vi "InjA-Image-RT.vi"() -> ()   [LabVIEW 2016]
uses:
  Common-Control/Cryo Readback.ctl
  Common-Control/Aperture states.ctl
  Common-Control/Faraday cup states.ctl
  Common-Control/GV states.ctl
  Common-Control/GP307 cluster.ctl
  <vilib>/userdefined/High Color/nirio_resource_hc.ctl
  Common-Control/Glassman Control.ctl
  <vilib>/FPGAPlugInAG/cRIO-9074/niLvFpga_Open_cRIO-9074.vi
  <vilib>/Utility/error.llb/Error Cluster From Error Code.vi
  <vilib>/rvi/errors/niLvFpgaAdjustHostInterfaceError.vi
  <vilib>/functionblocks/Control/PID/PID.vi
  <vilib>/rvi/interface/nirviOpenFPGA/nirviOpenFPGA.xnode
  FPGA Bitfiles/Controlsoftware2_FPGATarget_InjFPGA_-aTnSXeY2bA.lvbitx
  InjA-Image-FPGA.vi
  <vilib>/rvi/interface/nirviReadWriteControl/nirviReadWriteControl.xnode
  Common-Control/Faraday Cup Readback.ctl
  Common-Control/Aperture Readback.ctl
  Common-Control/Gate Valve Readback.ctl
  <vilib>/functionblocks/FB Core/FB Core.xnode
  <vilib>/functionblocks/FB Property/FB Overlay DBL.ctl
  <vilib>/functionblocks/NI_FunctionBlock Libraries.lvlib
  NiFpgaLv.dll
panel:
  out "Injector A Vac Interlock Bypass":bool
  out "Injector A Vac Interlock":bool
  out "Error Reporter":errorcluster
  in  "Tab Control":T1(tab)
  out "X-I":fxp<+/-,16,5>=1.28955078125
  out "X- V":fxp<+/-,16,5>=5.3388671875
  out "X+ I":fxp<+/-,16,5>=1.1064453125
  out "X+ V":fxp<+/-,16,5>=4.63671875
  out "Y+ V":fxp<+/-,16,5>=4.380859375
  out "Y+I":fxp<+/-,16,5>=1.068359375
  out "Y-V":fxp<+/-,16,5>=5.595703125
  out "Y-I":fxp<+/-,16,5>=1.36572265625
  out "Pre-acc V":fxp<+/-,16,5>=8.2509765625
  out "Pre-acc I":fxp<+/-,16,5>=2.544921875
  out "Einzel V":fxp<+/-,16,5>=7.4140625
  out "Einzel I":fxp<+/-,16,5>=1.6787109375
  out "X- Steerer Voltage Set":dbl
  out "X- Steerer HV Enable":bool
  out "X+ Steerer HV Enable":bool
  out "X+ Steerer Voltage Set":dbl
  out "Y- Steerer voltage set":dbl
  out "Y- Steerer HV Enable":bool
  out "Y+ Steerer HV Enable":bool
  out "Y+ Steerer voltage set":dbl
  out "Pre-Acc V set":dbl
  out "Pre-Acc HV Enable":bool
  out "Einzel HV Enable":bool
  out "Einzel V set":dbl
  in  "output low - switch":dbl
  in  "output high - switch":dbl=250.0
  out "Injector mag field set":dbl
  out "Injector mag field read 2":u8[](array[numeric])
  out "Injector mag field read":dbl
  out "Injector mag ps command":u8[](array[numeric])
  in  "derivative time (Td, min) - injector":dbl=0.01
  in  "integral time (Ti, min) - injector":dbl=0.01
  in  "proportional gain (Kc) - injector":dbl=10.0
  out "Injector mag command string":string
  out "Cryo Readback":T2
  out "Status":string
  out "On-time":string
  out "1st Stage Temp":string
  out "2nd Stage Temp":string
  out "Time since re-purge":string
  out "LowEnd Waist Vac Interlock":bool
  out "LowEnd Waist Vac Interlock bypass":bool
  out "Vac Interlock":bool
  out "Time since repurge":u8[](array[numeric])
  out "2nd stage temp":u8[](array[numeric])
  out "Cryo 1st stage temp":u8[](array[numeric])
  out "Cryo On-time":u8[](array[numeric])
  out "Cryo status":u8[](array[numeric])
  out "InjA Image Interlock bypass":bool
  out "Convectron 2":u8[](array[numeric])
  out "Ion Gauge 2":u8[](array[numeric])
  out "InjA Image Ion Gauge 1":dbl
  out "InjA Image Vac Cluster":T3
  out "InjA Image Convectron 1":dbl
  out "Convectron 1":u8[](array[numeric])
  out "Ion Gauge 1":u8[](array[numeric])
  out "Inj Image Aperture actuator":bool
  out "Inj Image FC actuator":bool
  out "Cryo Pump GV actuator":bool
  out "Beamline GV actuator":bool
  out "Inj Image Image  Aperture Position 2":T4
  out "Inj Image Image  Aperture Position":cluster{"IN sensor":bool, "OUT sensor":bool}
  out "Inj Image FC Status":T5
  out "Inj Image FC Position":cluster{"IN sensor":bool, "OUT sensor":bool}
  out "Beamline GV status":T6
  out "Beamline GV Position":T7
  out "Cryo Pump GV status":T6
  out "Cryo Pump GV Position":T7
  out "HV control loop error":errorcluster
  out "HV Readback loop error":errorcluster
  out "Injector Magnet error":errorcluster
  out "Cryo loop error":errorcluster
  out "GV Interlock loop error":errorcluster
  out "Acuator-Sensor loop error":errorcluster
  out "Vac cluster loop error":errorcluster
  in  "error in":errorcluster
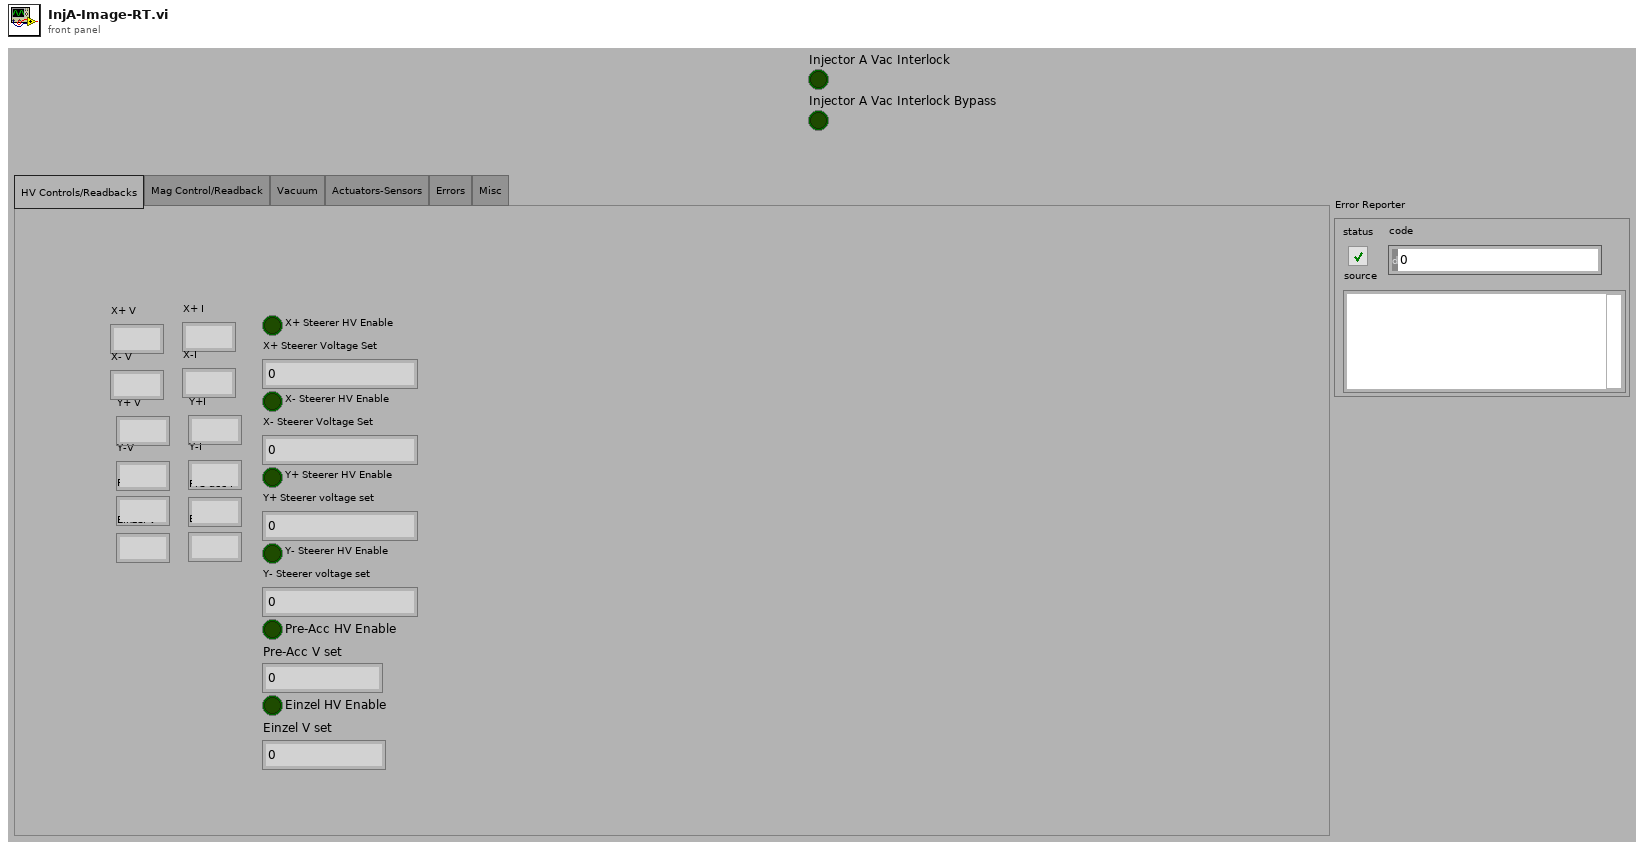
[diagram p1: front panel]
types:
  T1 = enum32{"HV Controls/Readbacks", "Mag Control/Readback", "Vacuum", "Actuators-Sensors", "Errors", "Misc"}
  T2 = typedef "Cryo Readback.ctl" = cluster{"Status":string, "On-time":string, "1st Stage Temp":string, "2nd Stage Temp":string, "Time since re-purge":string}
  T3 = typedef "GP307 cluster.ctl" = cluster{"Ion gauge 1":string, "Convectron  Gauge 1 ":string, "Ion Gauge 2":string, "Convectrom Gauge 2":string}
  T4 = typedef "Aperture states.ctl" = enum16{"Aperture status unclear", "Aperture in", "Aperture out"}
  T5 = typedef "Faraday cup states.ctl" = enum16{"FC status unclear", "FC in", "FC out"}
  T6 = typedef "GV states.ctl" = enum16{"status unclear", "closed", "open"}
  T7 = cluster{"OPEN sensor":bool, "Closed sensor":bool}
  T8 = typedef "nirio_resource_hc.ctl" = tag
  T9 = typedef "Faraday Cup Readback.ctl" = cluster{"IN sensor":bool, "OUT sensor":bool}
  T10 = typedef "Aperture Readback.ctl" = cluster{"IN sensor":bool, "OUT sensor":bool}
  T11 = typedef "Gate Valve Readback.ctl" = cluster{"OPEN sensor":bool, "Closed sensor":bool}
  T12 = typedef "Glassman Control.ctl" = cluster{"V-program":fxp<+/-,16,5>, "HV Enable":bool}
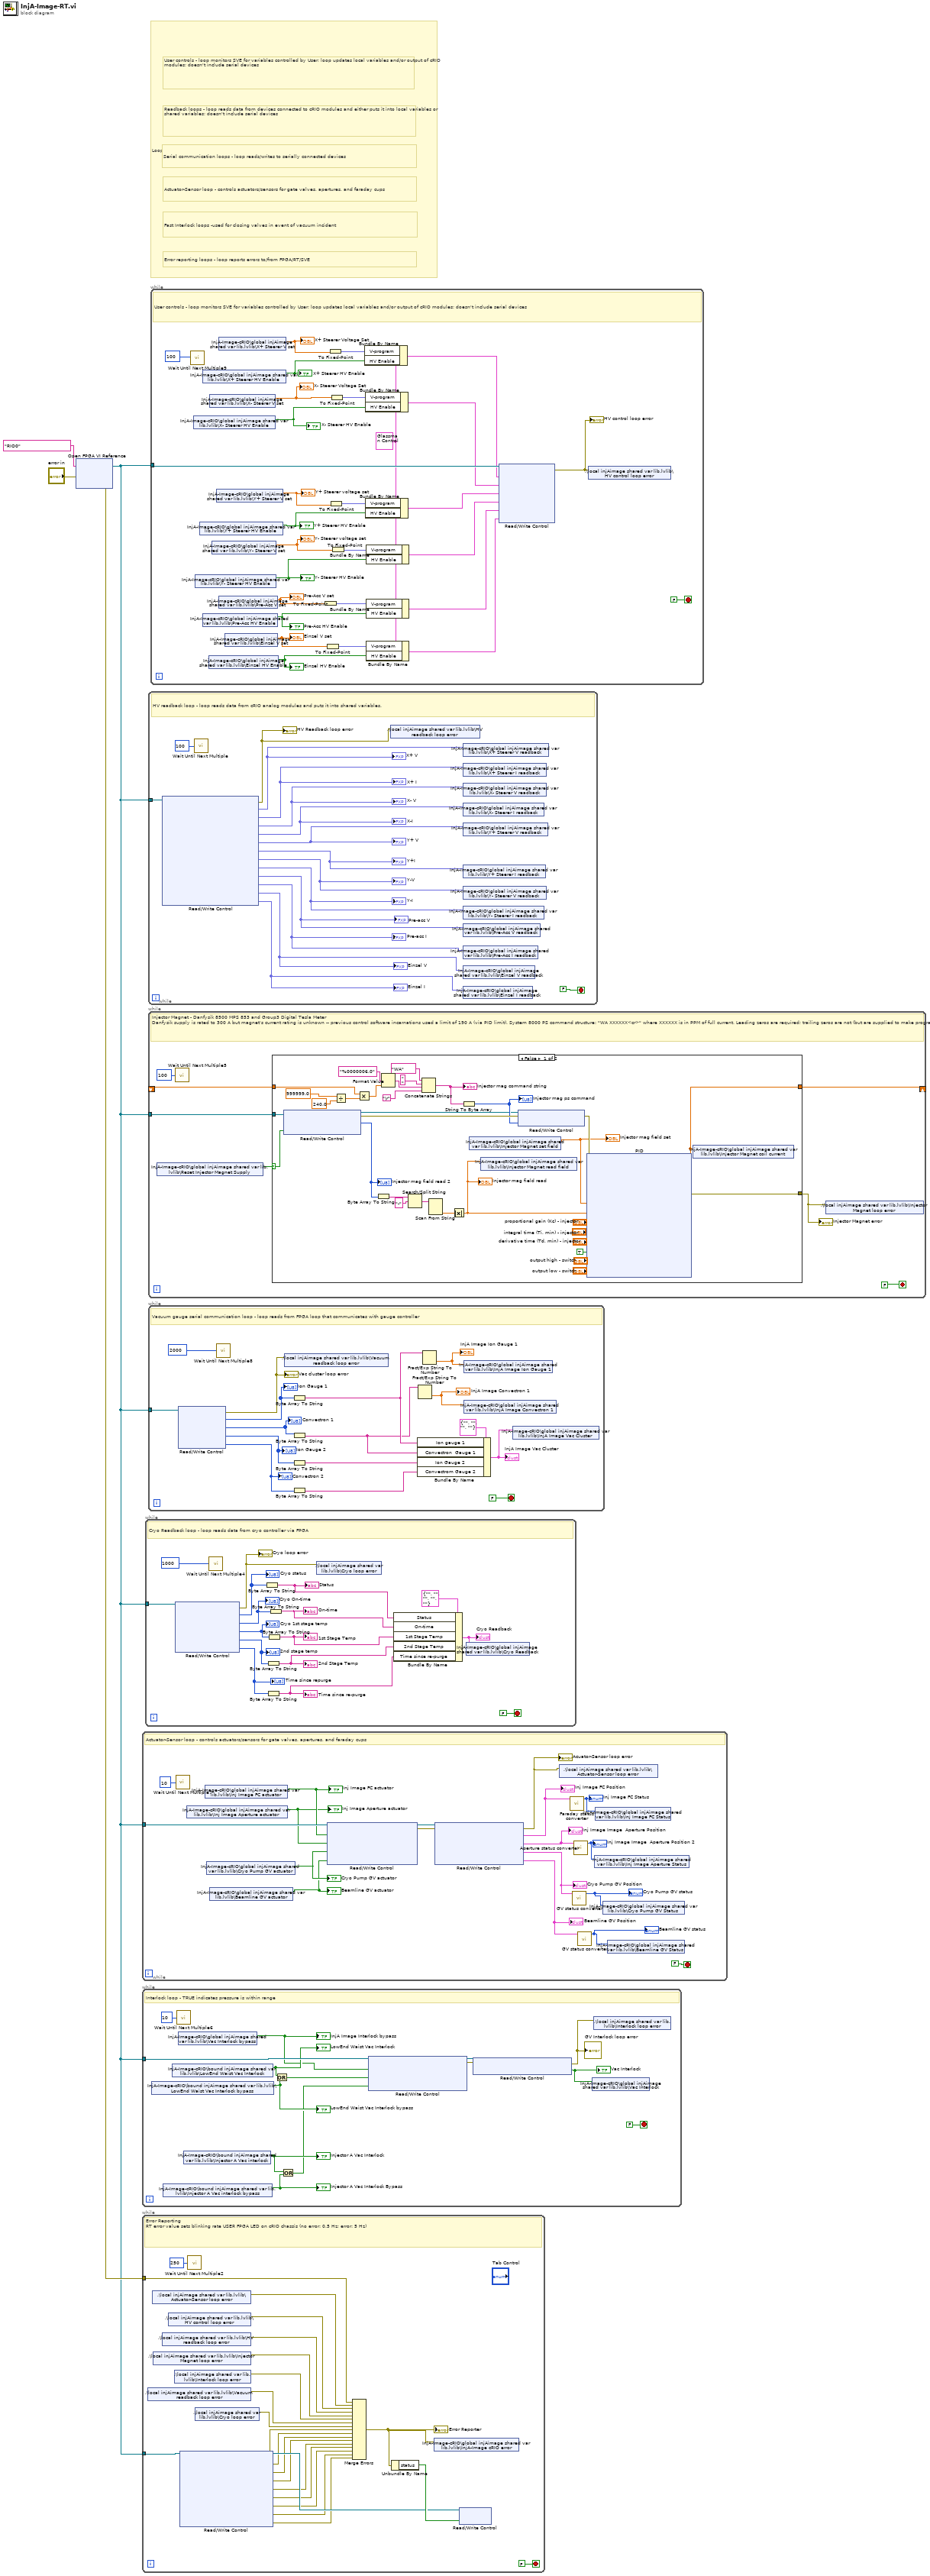
[diagram p0: block diagram]
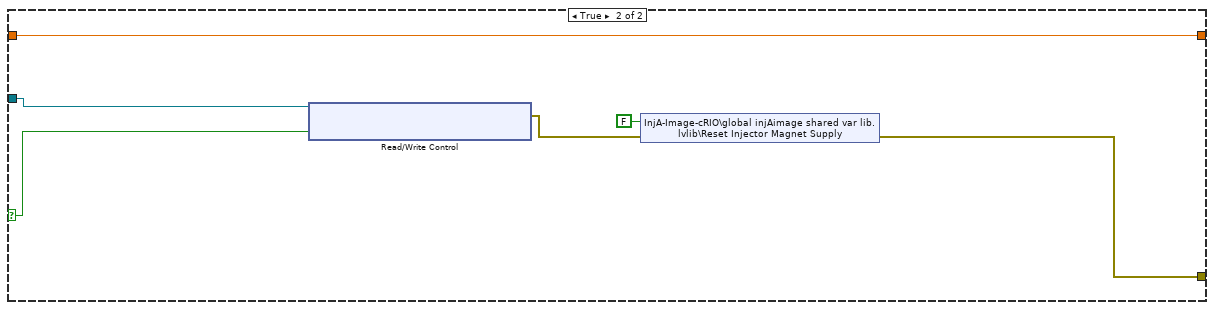
[diagram p2: hidden frame]
diagram:
  # "Serial communication loops - loop reads/writes to serially connected devices"
  # "Actuator-Sensor loop - controls actuators/sensors for gate valves, apertures, and faraday cups"
  # "Fast Interlock loops -used for closing valves in event of vacuum incident"
  # "Error reporting loops - loop reports errors to/from FPGA/RT/SVE"
  # "Readback loops - loop reads data from devices connected to cRIO modules and either puts it into local variables or shared variables; doesn't include serial devices"
  # "User controls - loop monitors SVE for variables controlled by User; loop updates local variables and/or output of cRIO modules; doesn't include serial devices"
  # "Loop legend - loops are color coded by responsibility"
  n1 = xnode "Open FPGA VI Reference"("error in"="error in", "resource name"=T8 "RIO0") -> ("FPGA VI Reference Out"=w1:refnum<k20>, "error out"=w2:errorcluster)
  n2 = while {
    tunnel: w1 -> [w22]
    stop <- FALSE stop-if-true
    # "Actuator-Sensor loop - controls actuators/sensors for gate valves, apertures, and faraday cups"
    n3 = call "Wait Until Next Multiple7"("Count(mSec)"=u32 10) -> ()  [unwired: 1 out]
    n4 = shared-variable "InjA-Image-cRIO\\global injAimage shared var lib.lvlib\\Inj Image Aperture actuator"() -> (w8:bool)  [unwired: 1 in, 1 out]
    "Inj Image Aperture actuator" <- w8
    n5 = shared-variable "InjA-Image-cRIO\\global injAimage shared var lib.lvlib\\Inj Image FC actuator"() -> (w9:bool)  [unwired: 1 in, 1 out]
    "Inj Image FC actuator" <- w9
    n6 = shared-variable "InjA-Image-cRIO\\global injAimage shared var lib.lvlib\\Cryo Pump GV actuator"() -> (w11:bool)  [unwired: 1 in, 1 out]
    "Cryo Pump GV actuator" <- w11
    n7 = shared-variable "InjA-Image-cRIO\\global injAimage shared var lib.lvlib\\Beamline GV actuator"() -> (w10:bool)  [unwired: 1 in, 1 out]
    "Beamline GV actuator" <- w10
    n8 = xnode "Read/Write Control"("FPGA VI Reference In"=w22, "Inj Image FC Actuator"=w9, "Inj Image Aperture Actuator"=w8, "Cryo Pump GV Actuator"=w11, "Beamline GV Actuator"=w10) -> ("FPGA VI Reference Out"=w20:refnum<k20>, "error out"=w18:errorcluster)  [unwired: 1 in]
    n9 = xnode "Read/Write Control"("FPGA VI Reference In"=w20, "error in"=w18) -> ("error out"=w12:errorcluster, "Inj Image FC Position"=w14:T9, "Inj Image Aperture Position"=w13:T10, "Cryo Pump GV Status"=w17:T11, "Beamline GV Status"=w16:T11)  [unwired: 1 out]
    "Cryo Pump GV Position" <- w17
    "Beamline GV Position" <- w16
    "Inj Image FC Position" <- w14
    "Inj Image Image  Aperture Position" <- w13
    "Acuator-Sensor loop error" <- w12
    n10 = shared-variable ".\\local injAimage shared var lib.lvlib\\Actuator-Sensor loop error"(w12) -> ()  [unwired: 1 in, 1 out]
    n11 = call "Faraday status converter.vi"("FC Position"=w14) -> ("FC Status"=w15:T5)  [unwired: 10 in]
    "Inj Image FC Status" <- w15
    n12 = call "GV status converter.vi"("Gate Valve"=w17) -> ("GV Status"=w6:T6)  [unwired: 10 in]
    "Cryo Pump GV status" <- w6
    n13 = call "Aperture status converter.vi"("Aperture Position"=w13) -> ("Aperture Status"=w5:T4)  [unwired: 10 in]
    "Inj Image Image  Aperture Position 2" <- w5
    n14 = call "GV status converter.vi"("Gate Valve"=w16) -> ("GV Status"=w7:T6)  [unwired: 10 in]
    "Beamline GV status" <- w7
    n15 = shared-variable "InjA-Image-cRIO\\global injAimage shared var lib.lvlib\\Inj Image Aperture Status"(w5) -> ()  [unwired: 1 in, 1 out]
    n16 = shared-variable "InjA-Image-cRIO\\global injAimage shared var lib.lvlib\\Inj Image FC Status"(w15) -> ()  [unwired: 1 in, 1 out]
    n17 = shared-variable "InjA-Image-cRIO\\global injAimage shared var lib.lvlib\\Cryo Pump GV Status"(w6) -> ()  [unwired: 1 in, 1 out]
    n18 = shared-variable "InjA-Image-cRIO\\global injAimage shared var lib.lvlib\\Beamline GV Status"(w7) -> ()  [unwired: 1 in, 1 out]
  }
  n19 = while {
    tunnel: w1 -> [w36]
    stop <- FALSE stop-if-true
    # "Interlock loop - TRUE indicates pressure is within range"
    n20 = shared-variable "InjA-Image-cRIO\\bound injAimage shared var lib.lvlib\\LowEnd Waist Vac Interlock bypass"() -> (w30:bool)  [unwired: 1 in, 1 out]
    "LowEnd Waist Vac Interlock bypass" <- w30
    n21 = shared-variable "InjA-Image-cRIO\\bound injAimage shared var lib.lvlib\\Injector A Vac interlock bypass"() -> (w25:bool)  [unwired: 1 in, 1 out]
    "Injector A Vac Interlock Bypass" <- w25
    n22 = shared-variable "InjA-Image-cRIO\\bound injAimage shared var lib.lvlib\\LowEnd Waist Vac Interlock"() -> (w28:bool)  [unwired: 1 in, 1 out]
    "LowEnd Waist Vac Interlock" <- w28
    n23 = call "Wait Until Next Multiple6"("Count(mSec)"=u32 10) -> ()  [unwired: 1 out]
    n24 = shared-variable "InjA-Image-cRIO\\global injAimage shared var lib.lvlib\\Vac Interlock bypass"() -> (w23:bool)  [unwired: 1 in, 1 out]
    "InjA Image Interlock bypass" <- w23
    n25 = shared-variable "InjA-Image-cRIO\\bound injAimage shared var lib.lvlib\\Injector A Vac interlock"() -> (w26:bool)  [unwired: 1 in, 1 out]
    "Injector A Vac Interlock" <- w26
    n26 = Or(x=w28, y=w30) -> (x .or. y?=w29:bool)
    n27 = Or(x=w26, y=w25) -> (x .or. y?=w24:bool)
    n28 = xnode "Read/Write Control"("FPGA VI Reference In"=w36, "Vac Interlock Bypass"=w23, "LowEnd Waist Vac Interlock"=w29, "InjectorA Vac Interlock"=w24) -> ("FPGA VI Reference Out"=w35:refnum<k20>, "error out"=w34:errorcluster)  [unwired: 1 in]
    n29 = xnode "Read/Write Control"("FPGA VI Reference In"=w35, "error in"=w34) -> ("error out"=w33:errorcluster, "Vac Interlock"=w27:bool)  [unwired: 1 out]
    "GV Interlock loop error" <- w33
    "Vac Interlock" <- w27
    n30 = shared-variable "InjA-Image-cRIO\\global injAimage shared var lib.lvlib\\Vac Interlock"(w27) -> ()  [unwired: 1 in, 1 out]
    n31 = shared-variable ".\\local injAimage shared var lib.lvlib\\Interlock loop error"(w33) -> ()  [unwired: 1 in, 1 out]
  }
  n32 = while {
    tunnel: w1 -> [w52]
    tunnel: w2 -> [w42]
    stop <- FALSE stop-if-true
    # "Error Reporting\nRT error value sets blinking rate USER FPGA LED on cRIO chassis (no error: 0.5 Hz; error: 5 Hz)"
    n33 = shared-variable ".\\local injAimage shared var lib.lvlib\\Vacuum readback loop error"() -> (w54:errorcluster)  [unwired: 1 in, 1 out]
    n34 = shared-variable ".\\local injAimage shared var lib.lvlib\\Actuator-Sensor loop error"() -> (w40:errorcluster)  [unwired: 1 in, 1 out]
    n35 = shared-variable ".\\local injAimage shared var lib.lvlib\\Injector Magnet loop error"() -> (w56:errorcluster)  [unwired: 1 in, 1 out]
    n36 = shared-variable ".\\local injAimage shared var lib.lvlib\\HV readback loop error"() -> (w57:errorcluster)  [unwired: 1 in, 1 out]
    n37 = shared-variable ".\\local injAimage shared var lib.lvlib\\HV control loop error"() -> (w41:errorcluster)  [unwired: 1 in, 1 out]
    n38 = shared-variable ".\\local injAimage shared var lib.lvlib\\Interlock loop error"() -> (w55:errorcluster)  [unwired: 1 in, 1 out]
    n39 = xnode "Read/Write Control"("FPGA VI Reference In"=w52) -> ("FPGA VI Reference Out"=w51:refnum<k20>, "error out"=w50:errorcluster, "GV Interlock loop error"=w49:errorcluster, "Actuator-Sensor Loop error"=w48:errorcluster, "Injector Hall Probe error"=w47:errorcluster, "Injector Magnet control error"=w46:errorcluster, "Vac readback loop error"=w45:errorcluster, "HV control loop error"=w44:errorcluster, "Cryo pump error"=w38:errorcluster, "HV Readback loop"=w37:errorcluster)  [unwired: 1 in]
    n40 = call "Wait Until Next Multiple2"("Count(mSec)"=u32 250 ("millisecond multiple")) -> ()  [unwired: 1 out]
    n41 = shared-variable ".\\local injAimage shared var lib.lvlib\\Cryo loop error"() -> (w53:errorcluster)  [unwired: 1 in, 1 out]
    n42 = Merge Errors(w42, w40, w41, w57, w56, w55, w54, w53, w50, w49, w48, w47, w46, w45, w44, w38, w37) -> (w59:errorcluster)
    "Error Reporter" <- w59
    n43 = Unbundle By Name(w59) -> ("status"=w58:bool)
    n44 = shared-variable "InjA-Image-cRIO\\global injAimage shared var lib.lvlib\\InjA-Image cRIO error"(w59) -> ()  [unwired: 1 in, 1 out]
    n45 = xnode "Read/Write Control"("FPGA VI Reference In"=w51, "RT error"=w58) -> ()  [unwired: 1 in, 2 out]
  }
  n46 = while {
    tunnel: w1 -> [w74]
    stop <- FALSE stop-if-true
    # "Cryo Readback loop - loop reads data from cryo controller via FPGA"
    n47 = xnode "Read/Write Control"("FPGA VI Reference In"=w74) -> ("error out"=w60:errorcluster, "Cryo status"=w71:u8[], "Cryo On-time"=w72:u8[], "1st stage temp"=w73:u8[], "2nd stage temp"=w70:u8[], "Time since repurge"=w69:u8[])  [unwired: 1 in, 1 out]
    "Cryo status" <- w71
    "Cryo On-time" <- w72
    "Cryo 1st stage temp" <- w73
    "Cryo loop error" <- w60
    "2nd stage temp" <- w70
    "Time since repurge" <- w69
    n48 = call "Wait Until Next Multiple4"("Count(mSec)"=u32 1000 ("millisecond multiple")) -> ()  [unwired: 1 out]
    n49 = Byte Array To String(unsigned byte array=w71) -> (string=w65:string)
    "Status" <- w65
    n50 = Byte Array To String(unsigned byte array=w70) -> (string=w62:string)
    "2nd Stage Temp" <- w62
    n51 = Byte Array To String(unsigned byte array=w69) -> (string=w61:string)
    "Time since re-purge" <- w61
    n52 = Byte Array To String(unsigned byte array=w73) -> (string=w63:string)
    "1st Stage Temp" <- w63
    n53 = Byte Array To String(unsigned byte array=w72) -> (string=w64:string)
    "On-time" <- w64
    n54 = shared-variable ".\\local injAimage shared var lib.lvlib\\Cryo loop error"(w60) -> ()  [unwired: 1 in, 1 out]
    n55 = Bundle By Name(cluster=T2 {"Status"="", "On-time"="", "1st Stage Temp"="", "2nd Stage Temp"="", "Time since re-purge"=""} ("Cryo Readback"), "Status"=w65, "On-time"=w64, "1st Stage Temp"=w63, "2nd Stage Temp"=w62, "Time since re-purge"=w61) -> (w67:T2)
    "Cryo Readback" <- w67
    n56 = shared-variable "InjA-Image-cRIO\\global injAimage shared var lib.lvlib\\Cryo Readback"(w67) -> ()  [unwired: 1 in, 1 out]
  }
  n57 = while {
    shift-right: [w78] -> _
    shift-left: _ -> [w80]
    tunnel: w1 -> [w81]
    stop <- FALSE stop-if-true
    # "Injector Magnet - Danfysik 8500 MPS 853 and Group3 Digital Tesla Meter\nDanfysik supply is rated to 300 A but magnet's current rating is unknown -- previous control software incarnations used a limit of 190 A (via PID limit). System 8000 PS command structure: \"WA XXXXXX<cr>\" where XXXXXX is in PPM of full current. Leading zeros are required; trailing zeros are not (but are supplied to make programming easier)"
    n58 = shared-variable "InjA-Image-cRIO\\global injAimage shared var lib.lvlib\\Reset Injector Magnet Supply"() -> (w77:bool)  [unwired: 1 in, 1 out]
    n59 = call "Wait Until Next Multiple5"("Count(mSec)"=u32 100 ("millisecond multiple")) -> ()  [unwired: 1 out]
    n60 = case shown="False" w77 {
      selector: w77 -> [w85 w184]
      tunnel: w81 -> [w101 w186]
      tunnel: w80 -> [w97 w185]
      tunnel: [w86 w185] -> w78
      tunnel: [w84 w181] -> w76
      frame False {
        n61 = xnode "Read/Write Control"("FPGA VI Reference In"=w101, "Inj Magnet Reset"=w85) -> ("FPGA VI Reference Out"=w95:refnum<k20>, "error out"=w100:errorcluster, "Injector Mag Field read"=w96:u8[])  [unwired: 1 in]
        "Injector mag field read 2" <- w96
        n62 = Divide(x=999999.0 ("y"), y=240.0) -> (x/y=w89:dbl)
        n63 = Multiply(x=w97, y=w89) -> (x*y=w110:dbl)
        n64 = Byte Array To String(unsigned byte array=w96) -> (string=w107:string)
        n65 = Format Value(format string="%0000006.0", value (0)=w110) -> (output string=w113:string)  [unwired: 1 out]
        n66 = Search/Split String(string=w107, search string/char (-)="-") -> (match + rest of string=w98:string)  [unwired: 3 out]
        n67 = Concatenate Strings("WA", " ", w113, "\r") -> (w114:string)
        "Injector mag command string" <- w114
        n68 = Scan From String(input string=w98) -> (output 1=w106:dbl)  [unwired: 3 in, 4 out]
        n69 = Absolute Value(x=w106) -> (abs(x)=w83:dbl)
        "Injector mag field read" <- w83
        n70 = String To Byte Array(string=w114) -> (unsigned byte array=w99:u8[])
        "Injector mag ps command" <- w99
        n71 = shared-variable "InjA-Image-cRIO\\global injAimage shared var lib.lvlib\\Injector Magnet set field"() -> (w87:dbl)  [unwired: 1 in, 1 out]
        "Injector mag field set" <- w87
        n72 = shared-variable "InjA-Image-cRIO\\global injAimage shared var lib.lvlib\\Injector Magnet read field"(w83) -> ()  [unwired: 1 in, 1 out]
        n73 = xnode "Read/Write Control"("FPGA VI Reference In"=w95, "error in"=w100, "Injector Magnet Set"=w99) -> ("error out"=w94:errorcluster)  [unwired: 1 out]
        n74 = xnode "PID"("error in"=w94, "setpoint"=w87, "process variable"=w83, "proportional gain (Kc)"="proportional gain (Kc) - injector", "integral time (Ti, min)"="integral time (Ti, min) - injector", "derivative time (Td, min)"="derivative time (Td, min) - injector", "auto? (T)"=TRUE, "output high"="output high - switch", "output low"="output low - switch") -> ("error out"=w84:errorcluster, "output"=w86:dbl)
        n75 = shared-variable "InjA-Image-cRIO\\global injAimage shared var lib.lvlib\\Injector Magnet coil current"(w86) -> ()  [unwired: 1 in, 1 out]
      }
      frame True {
        n76 = xnode "Read/Write Control"("FPGA VI Reference In"=w186, "Inj Magnet Reset"=w184) -> ("error out"=w182:errorcluster)  [unwired: 1 in, 1 out]
        n77 = shared-variable "InjA-Image-cRIO\\global injAimage shared var lib.lvlib\\Reset Injector Magnet Supply"(FALSE ("Reset Injector Magnet Supply"), error in=w182) -> (error out=w181:errorcluster)
      }
    }
    "Injector Magnet error" <- w76
    n78 = shared-variable ".\\local injAimage shared var lib.lvlib\\Injector Magnet loop error"(w76) -> ()  [unwired: 1 in, 1 out]
  }
  n79 = while {
    tunnel: w1 -> [w197]
    stop <- FALSE stop-if-true
    # "Vacuum gauge serial communication loop - loop reads from FPGA loop that communicates with gauge controller"
    n80 = xnode "Read/Write Control"("FPGA VI Reference In"=w197) -> ("error out"=w192:errorcluster, "Ion gauge 1"=w198:u8[], "Convectron 1"=w194:u8[], "Ion gauge 2"=w199:u8[], "Convectron 2"=w200:u8[])  [unwired: 1 in, 1 out]
    "Ion Gauge 1" <- w198
    "Convectron 1" <- w194
    "Ion Gauge 2" <- w199
    "Convectron 2" <- w200
    "Vac cluster loop error" <- w192
    n81 = call "Wait Until Next Multiple8"("Count(mSec)"=u32 2000 ("millisecond multiple")) -> ()  [unwired: 1 out]
    n82 = shared-variable ".\\local injAimage shared var lib.lvlib\\Vacuum readback loop error"(w192) -> ()  [unwired: 1 in, 1 out]
    n83 = Byte Array To String(unsigned byte array=w198) -> (string=w195:string)
    n84 = Byte Array To String(unsigned byte array=w194) -> (string=w193:string)
    n85 = Byte Array To String(unsigned byte array=w199) -> (string=w201:string)
    n86 = Byte Array To String(unsigned byte array=w200) -> (string=w202:string)
    n87 = Bundle By Name(cluster=T3 {"Ion gauge 1"="", "Convectron  Gauge 1 "="", "Ion Gauge 2"="", "Convectrom Gauge 2"=""} ("Ion gauge cluster control"), "Ion gauge 1"=w195, "Convectron  Gauge 1"=w193, "Ion Gauge 2"=w201, "Convectrom Gauge 2"=w202) -> (w189:T3)
    "InjA Image Vac Cluster" <- w189
    n88 = Fract/Exp String To Number(string=w193) -> (number=w188:dbl)  [unwired: 3 in, 1 out]
    "InjA Image Convectron 1" <- w188
    n89 = Fract/Exp String To Number(string=w195) -> (number=w187:dbl)  [unwired: 3 in, 1 out]
    "InjA Image Ion Gauge 1" <- w187
    n90 = shared-variable "InjA-Image-cRIO\\global injAimage shared var lib.lvlib\\InjA Image Ion Gauge 1"(w187) -> ()  [unwired: 1 in, 1 out]
    n91 = shared-variable "InjA-Image-cRIO\\global injAimage shared var lib.lvlib\\InjA Image Convectron 1"(w188) -> ()  [unwired: 1 in, 1 out]
    n92 = shared-variable "InjA-Image-cRIO\\global injAimage shared var lib.lvlib\\InjA Image Vac Cluster"(w189) -> ()  [unwired: 1 in, 1 out]
  }
  n93 = while {
    tunnel: w1 -> [w204]
    stop <- FALSE stop-if-true
    # "HV readback loop - loop reads data from cRIO analog modules and puts it into shared variables."
    n94 = xnode "Read/Write Control"("FPGA VI Reference In"=w204) -> ("error out"=w203:errorcluster, "X+ Steerer Monitor.I-monitor"=w216:fxp<+/-,16,5>, "X+ Steerer Monitor.V-monitor"=w215:fxp<+/-,16,5>, "X- Steerer Monitor.I-monitor"=w214:fxp<+/-,16,5>, "X- Steerer Monitor.V-monitor"=w213:fxp<+/-,16,5>, "Y+ Steerer Monitor.I-monitor"=w212:fxp<+/-,16,5>, "Y+ Steerer Monitor.V-monitor"=w205:fxp<+/-,16,5>, "Y- Steerer Monitor.I-monitor"=w206:fxp<+/-,16,5>, "Y- Steerer Monitor.V-monitor"=w207:fxp<+/-,16,5>, "Pre-Acc Monitor.I-monitor"=w208:fxp<+/-,16,5>, "Pre-Acc Monitor.V-monitor"=w209:fxp<+/-,16,5>, "Einzel Monitor.I-monitor"=w210:fxp<+/-,16,5>, "Einzel Monitor.V-monitor"=w211:fxp<+/-,16,5>)  [unwired: 1 in, 1 out]
    "Y+ V" <- w212
    "Y+I" <- w205
    "Y-V" <- w206
    "Y-I" <- w207
    "Pre-acc V" <- w208
    "Pre-acc I" <- w209
    "Einzel V" <- w210
    "Einzel I" <- w211
    "X+ V" <- w216
    "X+ I" <- w215
    "X- V" <- w214
    "X-I" <- w213
    "HV Readback loop error" <- w203
    n95 = call "Wait Until Next Multiple"("Count(mSec)"=u32 100) -> ()  [unwired: 1 out]
    n96 = shared-variable ".\\local injAimage shared var lib.lvlib\\HV readback loop error"(w203) -> ()  [unwired: 1 in, 1 out]
    n97 = shared-variable "InjA-Image-cRIO\\global injAimage shared var lib.lvlib\\X+ Steerer V readback"(w216) -> ()  [unwired: 1 in, 1 out]
    n98 = shared-variable "InjA-Image-cRIO\\global injAimage shared var lib.lvlib\\X+ Steerer I readback"(w215) -> ()  [unwired: 1 in, 1 out]
    n99 = shared-variable "InjA-Image-cRIO\\global injAimage shared var lib.lvlib\\X- Steerer V readback"(w214) -> ()  [unwired: 1 in, 1 out]
    n100 = shared-variable "InjA-Image-cRIO\\global injAimage shared var lib.lvlib\\X- Steerer I readback"(w213) -> ()  [unwired: 1 in, 1 out]
    n101 = shared-variable "InjA-Image-cRIO\\global injAimage shared var lib.lvlib\\Y+ Steerer V readback"(w212) -> ()  [unwired: 1 in, 1 out]
    n102 = shared-variable "InjA-Image-cRIO\\global injAimage shared var lib.lvlib\\Y+ Steerer I readback"(w205) -> ()  [unwired: 1 in, 1 out]
    n103 = shared-variable "InjA-Image-cRIO\\global injAimage shared var lib.lvlib\\Y- Steerer V readback"(w206) -> ()  [unwired: 1 in, 1 out]
    n104 = shared-variable "InjA-Image-cRIO\\global injAimage shared var lib.lvlib\\Y- Steerer I readback"(w207) -> ()  [unwired: 1 in, 1 out]
    n105 = shared-variable "InjA-Image-cRIO\\global injAimage shared var lib.lvlib\\Pre-Acc V readback"(w208) -> ()  [unwired: 1 in, 1 out]
    n106 = shared-variable "InjA-Image-cRIO\\global injAimage shared var lib.lvlib\\Pre-Acc I readback"(w209) -> ()  [unwired: 1 in, 1 out]
    n107 = shared-variable "InjA-Image-cRIO\\global injAimage shared var lib.lvlib\\Einzel V readback"(w210) -> ()  [unwired: 1 in, 1 out]
    n108 = shared-variable "InjA-Image-cRIO\\global injAimage shared var lib.lvlib\\Einzel I readback"(w211) -> ()  [unwired: 1 in, 1 out]
  }
  n109 = while {
    tunnel: w1 -> [w247]
    stop <- FALSE stop-if-true
    w227 = T12 {"V-program"=0.0, "HV Enable"=FALSE} ("Glassman Control")
    # "User controls - loop monitors SVE for variables controlled by User; loop updates local variables and/or output of cRIO modules; doesn't include serial devices"
    n110 = call "Wait Until Next Multiple9"("Count(mSec)"=u32 100 ("millisecond multiple")) -> ()  [unwired: 1 out]
    n111 = shared-variable "InjA-Image-cRIO\\global injAimage shared var lib.lvlib\\X- Steerer HV Enable"() -> (w233:bool)  [unwired: 1 in, 1 out]
    "X- Steerer HV Enable" <- w233
    n112 = shared-variable "InjA-Image-cRIO\\global injAimage shared var lib.lvlib\\Y- Steerer HV Enable"() -> (w229:bool)  [unwired: 1 in, 1 out]
    "Y- Steerer HV Enable" <- w229
    n113 = shared-variable "InjA-Image-cRIO\\global injAimage shared var lib.lvlib\\Y+ Steerer HV Enable"() -> (w231:bool)  [unwired: 1 in, 1 out]
    "Y+ Steerer HV Enable" <- w231
    n114 = shared-variable "InjA-Image-cRIO\\global injAimage shared var lib.lvlib\\X+ Steerer HV Enable"() -> (w236:bool)  [unwired: 1 in, 1 out]
    "X+ Steerer HV Enable" <- w236
    n115 = shared-variable "InjA-Image-cRIO\\global injAimage shared var lib.lvlib\\Pre-Acc HV Enable"() -> (w221:bool)  [unwired: 1 in, 1 out]
    "Pre-Acc HV Enable" <- w221
    n116 = shared-variable "InjA-Image-cRIO\\global injAimage shared var lib.lvlib\\Einzel HV Enable"() -> (w223:bool)  [unwired: 1 in, 1 out]
    "Einzel HV Enable" <- w223
    n117 = shared-variable "InjA-Image-cRIO\\global injAimage shared var lib.lvlib\\X- Steerer V set"() -> (w234:dbl)  [unwired: 1 in, 1 out]
    "X- Steerer Voltage Set" <- w234
    n118 = shared-variable "InjA-Image-cRIO\\global injAimage shared var lib.lvlib\\Y- Steerer V set"() -> (w230:dbl)  [unwired: 1 in, 1 out]
    "Y- Steerer voltage set" <- w230
    n119 = shared-variable "InjA-Image-cRIO\\global injAimage shared var lib.lvlib\\Y+ Steerer V set"() -> (w232:dbl)  [unwired: 1 in, 1 out]
    "Y+ Steerer voltage set" <- w232
    n120 = shared-variable "InjA-Image-cRIO\\global injAimage shared var lib.lvlib\\X+ Steerer V set"() -> (w235:dbl)  [unwired: 1 in, 1 out]
    "X+ Steerer Voltage Set" <- w235
    n121 = shared-variable "InjA-Image-cRIO\\global injAimage shared var lib.lvlib\\Pre-Acc V set"() -> (w222:dbl)  [unwired: 1 in, 1 out]
    "Pre-Acc V set" <- w222
    n122 = shared-variable "InjA-Image-cRIO\\global injAimage shared var lib.lvlib\\Einzel V set"() -> (w224:dbl)  [unwired: 1 in, 1 out]
    "Einzel V set" <- w224
    n123 = To Fixed-Point(number=w222) -> (fixed-point=w220:fxp<+/-,16,5>)  [unwired: 1 in]
    n124 = To Fixed-Point(number=w224) -> (fixed-point=w219:fxp<+/-,16,5>)  [unwired: 1 in]
    n125 = To Fixed-Point(number=w235) -> (fixed-point=w240:fxp<+/-,20,5>)  [unwired: 1 in]
    n126 = To Fixed-Point(number=w232) -> (fixed-point=w244:fxp<+/-,16,5>)  [unwired: 1 in]
    n127 = To Fixed-Point(number=w234) -> (fixed-point=w239:fxp<+/-,16,5>)  [unwired: 1 in]
    n128 = To Fixed-Point(number=w230) -> (fixed-point=w243:fxp<+/-,16,5>)  [unwired: 1 in]
    n129 = Bundle By Name(cluster=w227, "V-program"=w240, "HV Enable"=w236) -> (w237:T12)
    n130 = Bundle By Name(cluster=w227, "V-program"=w239, "HV Enable"=w233) -> (w238:T12)
    n131 = Bundle By Name(cluster=w227, "V-program"=w244, "HV Enable"=w231) -> (w241:T12)
    n132 = Bundle By Name(cluster=w227, "V-program"=w243, "HV Enable"=w229) -> (w242:T12)
    n133 = Bundle By Name(cluster=w227, "V-program"=w220, "HV Enable"=w221) -> (w226:T12)
    n134 = Bundle By Name(cluster=w227, "V-program"=w219, "HV Enable"=w223) -> (w225:T12)
    n135 = xnode "Read/Write Control"("FPGA VI Reference In"=w247, "X+ Steerer V set"=w237, "X- Steerer V set"=w238, "Y+ Steerer V set"=w241, "Y- Steerer V set"=w242, "Pre-Acc V set"=w226, "Einzel V set"=w225) -> ("error out"=w245:errorcluster)  [unwired: 1 in, 1 out]
    "HV control loop error" <- w245
    n136 = shared-variable ".\\local injAimage shared var lib.lvlib\\HV control loop error"(w245) -> ()  [unwired: 1 in, 1 out]
  }
